vi "TL_save_path_definition.vi"(3 "error in":errorcluster, 4 "Sample name":string, 5 "Path to the saving folder":path) -> (0 "error out":errorcluster, 1 "TL movie path":path, 2 "TL path":path)   [LabVIEW 2015]
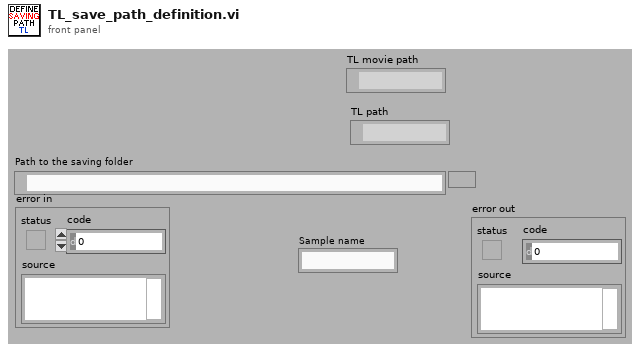
[diagram p1: front panel]
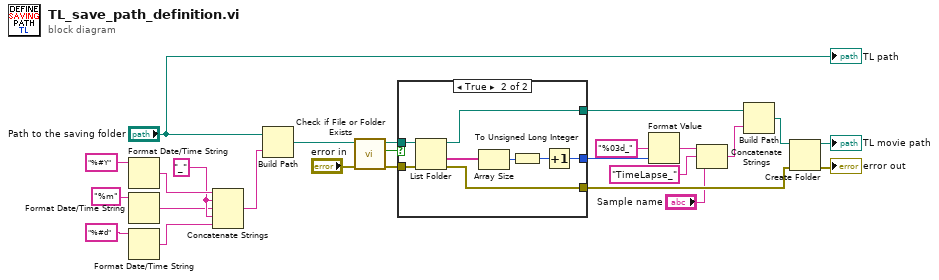
[diagram p0: block diagram]
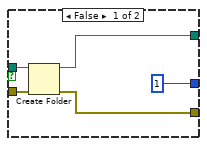
[diagram p2: hidden frame]
diagram:
  w23 = "_" ("string")
  n1 = Format Date/Time String(time format string (%c)="%#Y") -> (date/time string=w24:string)  [unwired: 2 in]
  n2 = Format Date/Time String(time format string (%c)="%m") -> (date/time string=w20:string)  [unwired: 2 in]
  n3 = Format Date/Time String(time format string (%c)="%#d") -> (date/time string=w19:string)  [unwired: 2 in]
  n4 = Concatenate Strings(w24, w23, w20, w23, w19) -> (w18:string)
  n5 = Build Path(base path="Path to the saving folder", name or relative path=w18) -> (appended path=w17:path)
  n6 = call <vilib>:"Check if File or Folder Exists.vi"("error in (no error)"="error in", "path"=w17) -> ("error out"=w5:errorcluster, "file or folder exists?"=w6:bool, "dup path"=w7:path)  [unwired: 7 in]
  n7 = case shown="True" w6 {
    tunnel: w5 -> [w30 w38]
    tunnel: w7 -> [w29 w37]
    tunnel: [w28 w36] -> w8
    tunnel: [w27 w35] -> w15
    tunnel: [u32 1 w32] -> w13
    frame False {
      n8 = Create Folder(path (use dialog)=w29, error in=w30) -> (created path=w27:path, error out=w28:errorcluster)  [unwired: 1 in, 1 out]
    }
    frame True {
      n9 = List Folder(path=w37, error in=w38) -> (path out=w35:path, folder names=w33:string[], error out=w36:errorcluster)  [unwired: 2 in, 1 out]
      n10 = Array Size(array=w33) -> (size(s)=w34:i32)
      n11 = To Unsigned Long Integer(number=w34) -> (unsigned 32bit integer=w31:u32)
      n12 = Increment(x=w31) -> (x+1=w32:u32)
    }
  }
  n13 = Format Value(format string="%03d_" ("string (\"\")"), value (0)=w13) -> (output string=w12:string)  [unwired: 1 in]
  n14 = Concatenate Strings(w12, "TimeLapse_" ("string"), "Sample name") -> (w10:string)
  n15 = Build Path(base path=w15, name or relative path=w10) -> (appended path=w9:path)
  n16 = Create Folder(path (use dialog)=w9, error in=w8) -> (created path=→"TL movie path":path, error out=→"error out":errorcluster)  [unwired: 1 in, 1 out]
  "TL path" <- "Path to the saving folder"
